vi "ROI-SelectionAndorNull.vi"(8 "error in (no error)":errorcluster, 9 "Global Rectangle":i32[](array[numeric]), 11 "Image In":i32[][](array[numeric])) -> (0 "error out":errorcluster, 2 "ROI Coordinates out":T1, 3 "Image Out":i32[][](array[numeric]))   [LabVIEW 2011]
panel:
  in  "ROI Coordinates out 2":T1
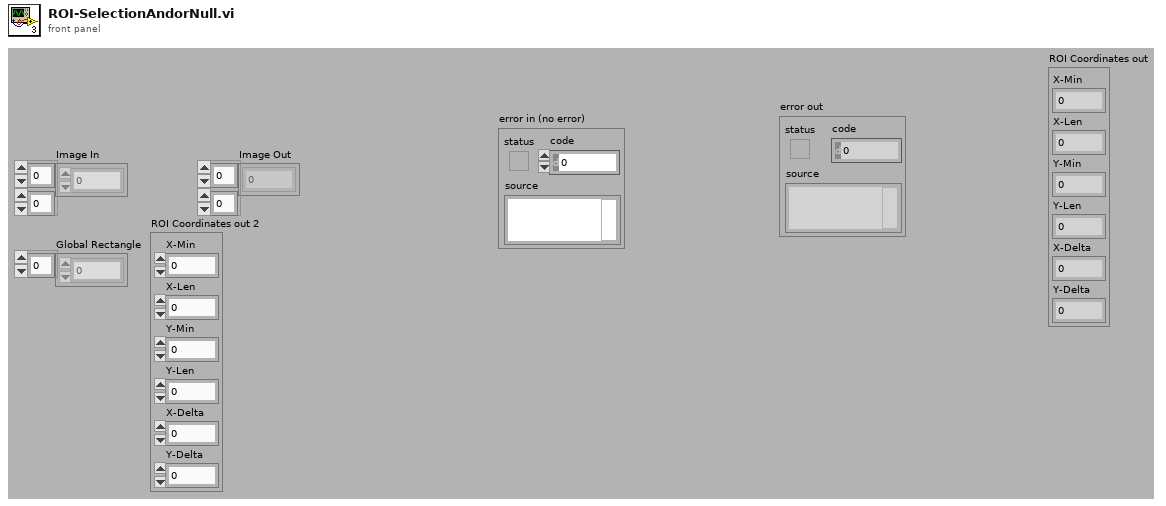
[diagram p1: front panel]
types:
  T1 = cluster{"X-Min":i32, "X-Len":i32, "Y-Min":i32, "Y-Len":i32, "X-Delta":i32, "Y-Delta ":i32}
  T2 = cluster{"X-Min":dbl, "X-Len":dbl, "Y-Min":dbl, "Y-Len":dbl, "X-Delta":dbl, "Y-Delta ":dbl}
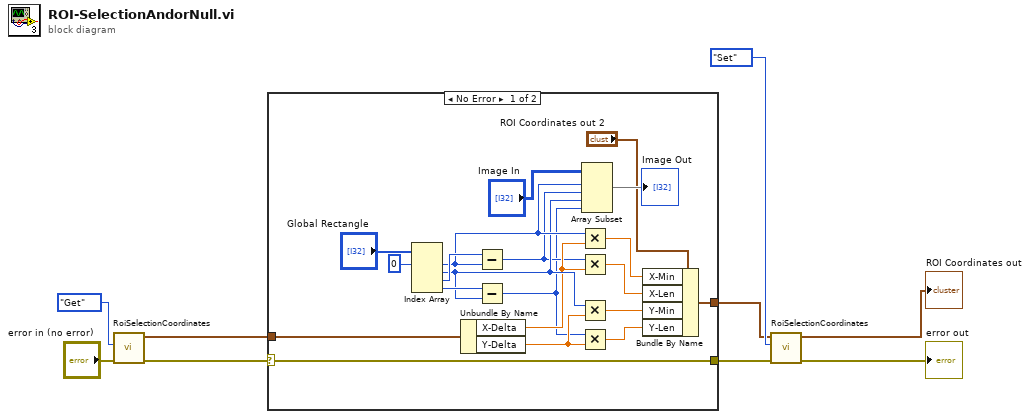
[diagram p0: block diagram]
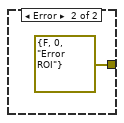
[diagram p2: hidden frame]
diagram:
  n1 = call "RoiSelectionCoordinates.vi"("error in"="error in (no error)", "FGV_Control"=enum16{"Set", "Get"}."Get") -> ("error out"=w3:errorcluster, "ROI Coordinates out"=w1:T2)  [unwired: 8 in]
  n2 = case shown="No Error" w3 {
    selector: w3 -> [w10 _]
    tunnel: [w10 errorcluster {"status"=FALSE, "code"=0, "source"="Error ROI"} ("error IO")] -> w5
    tunnel: [w23 _] -> w7
    tunnel: w1 -> [w11 _]
    frame No Error {
      n3 = Index Array(array="Global Rectangle", index #1=0 ("index")) -> (element #1=w21:i32, element #2=w19:i32, element #3=w26:i32, element #4=w27:i32)  [unwired: 3 in]
      n4 = Unbundle By Name(w11) -> ("X-Delta"=w17:dbl, "Y-Delta"=w16:dbl)
      n5 = Subtract(x=w26, y=w21) -> (x-y=w15:i32)
      n6 = Subtract(x=w27, y=w19) -> (x-y=w13:i32)
      n7 = Multiply(x=w21, y=w17) -> (x*y=w20:dbl)
      n8 = Multiply(x=w15, y=w17) -> (x*y=w14:dbl)
      n9 = Multiply(x=w19, y=w16) -> (x*y=w18:dbl)
      n10 = Multiply(x=w13, y=w16) -> (x*y=w12:dbl)
      n11 = Array Subset(array="Image In", index (row)=w21, length (row)=w15, index (col)=w19, length (col)=w13) -> (→"Image Out":i32[][])
      n12 = Bundle By Name(cluster="ROI Coordinates out 2", "X-Min"=w20, "X-Len"=w14, "Y-Min"=w18, "Y-Len"=w12) -> (w23:T1)
    }
    frame Error {
    }
  }
  n13 = call "RoiSelectionCoordinates.vi"("error in"=w5, "FGV_Control"=enum16{"Set", "Get"}."Set", "ROI Coordinates in"=w7) -> ("error out"=→"error out":errorcluster, "ROI Coordinates out"=→"ROI Coordinates out":T2)  [unwired: 7 in]
